vi "Keithley2450 DC Ramp to Block.vi"() -> ()   [LabVIEW 2020]
uses:
  <vilib>/Analysis/1siggen.llb/Ramp Pattern by Samples.vi
  <vilib>/Waveform/WDTOps.llb/WDT Append Waveforms DBL.vi
  <instrlib>/Keithley 2450/Public/Data/Read (Multiple Points).vi
  <vilib>/measure/NI_MAPro.lvlib
  <instrlib>/Keithley 2450/Keithley 2450.lvlib
  <vilib>/Analysis/NI_AALBase.lvlib
panel:
  in  "Source Mode":enum16{"Voltage", "Current"}(ring)=enum."Current"
  in  "VISA resource name":refnum<visa-resource-name>
  in  "Compliance\nVoltage":dbl=210.0
  out "Output Waveform":waveform(dbl)(graph)
  out "Total Time":dbl
  in  "End Amplitude\nHold Time (s)":dbl
  in  "End Amplitude\n(mU)":dbl
  in  "Ramp Rate\n(|mU/s|)":dbl
  in  "Start Amplitude\n(mU)":dbl
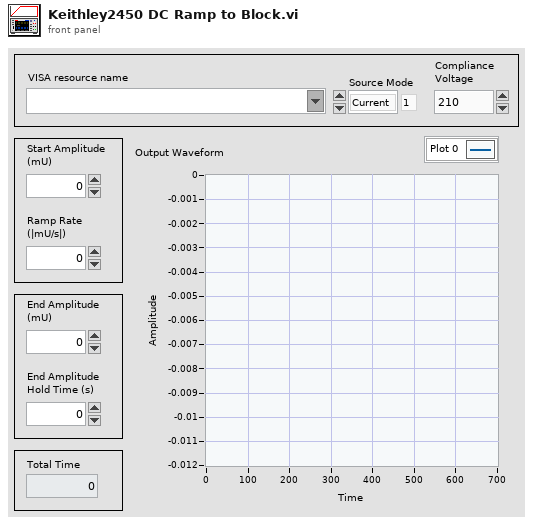
[diagram p1: front panel]
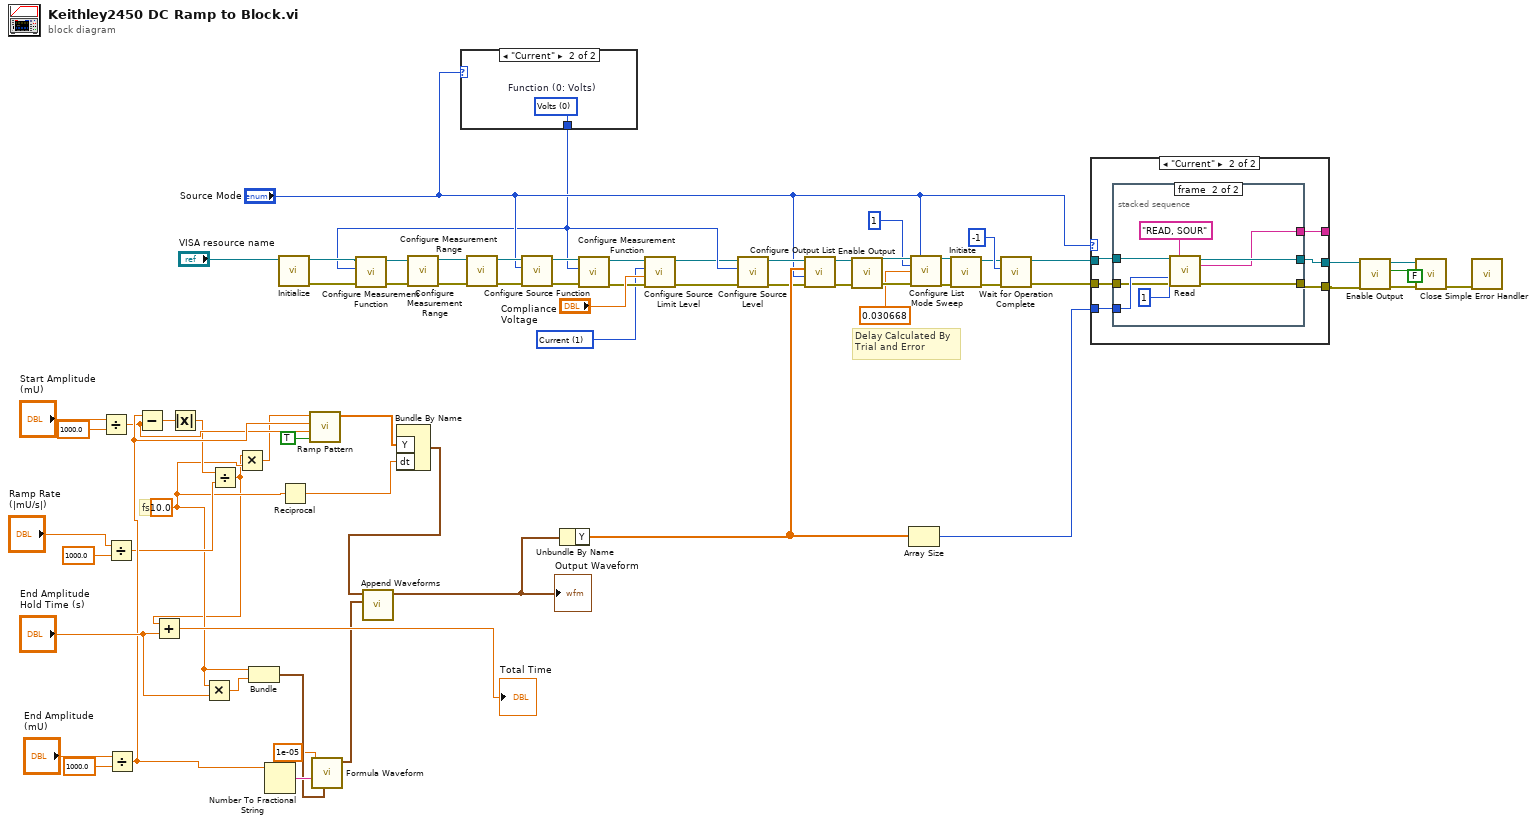
[diagram p0: block diagram]
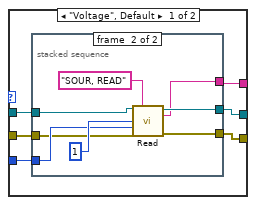
[diagram p2: hidden frame]
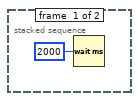
[diagram p3: hidden frame]
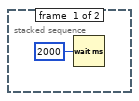
[diagram p4: hidden frame]
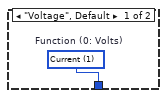
[diagram p5: hidden frame]
diagram:
  w24 = u16 1 items=["Volts", "Current"] ("Function (0: Volts)")
  w2 = 10.0
  # "Delay Calculated By\nTrial and Error"
  # "fs"
  n1 = Divide(x="Start Amplitude\n(mU)", y=1000.0) -> (x/y=w10:dbl)
  n2 = Divide(x="Ramp Rate\n(|mU/s|)", y=1000.0) -> (x/y=w8:dbl)
  n3 = Divide(x="End Amplitude\n(mU)", y=1000.0) -> (x/y=w11:dbl)
  n4 = Subtract(x=w11, y=w10) -> (x-y=w12:dbl)
  n5 = Absolute Value(x=w12) -> (abs(x)=w9:dbl)
  n6 = Multiply(x=w2, y="End Amplitude\nHold Time (s)") -> (x*y=w68:dbl)
  n7 = Divide(x=w9, y=w8) -> (x/y=w1:dbl)
  n8 = Add(x=w1, y="End Amplitude\nHold Time (s)") -> (x+y=→"Total Time":dbl)
  n9 = Multiply(x=w1, y=w2) -> (x*y=w7:dbl)
  n10 = Bundle(w2, w68) -> (w66:cluster{dbl, dbl})  [unwired: 1 in]
  n11 = Number To Fractional String(number=w11) -> (F-format string=w67:string)  [unwired: 3 in]
  n12 = call <instrlib>:"Initialize.vi"("VISA resource name"="VISA resource name") -> ("error out"=w52:errorcluster, "VISA resource name out"=w50:refnum<visa-resource-name>)  [unwired: 9 in]
  n13 = Reciprocal(x=w2) -> (1/x=w5:dbl)
  n14 = call-poly <vilib>:"Ramp Pattern.vi"("exclude end?"=TRUE, "start"=w10, "end"=w11, "samples"=w7) -> ("Ramp Pattern"=w6:dbl[])  [unwired: 6 in, 1 out]
  n15 = call <vilib>:"Formula Waveform.vi"("sampling info"=w66, "formula"=w67, "frequency"=1e-05) -> ("signal out"=w62:waveform(dbl))  [unwired: 7 in, 1 out]
  n16 = Bundle By Name("Y"=w6, "dt"=w5) -> (w4:waveform(dbl))  [unwired: 1 in]
  n17 = call-poly <vilib>:"Append Waveforms.vi"("waveform B"=w62, "waveform A"=w4) -> ("waveform out"=w61:waveform(dbl))  [unwired: 8 in, 1 out]
  "Output Waveform" <- w61
  n18 = case shown="\"Current\"" "Source Mode" {
    tunnel: [w69 w70] -> w25
    frame "Voltage", Default {
      w69 = u16 1 items=["Volts", "Current", "Resistance"]  # Function (0: Volts)
    }
    frame "Current" {
      w70 = u16 0 items=["Volts", "Current", "Resistance"]  # Function (0: Volts)
    }
  }
  n19 = call <instrlib>:"Configure Measurement Function.vi"("error in (no error)"=w52, "Function (0: Volts)"=w25, "VISA resource name"=w50) -> ("error out"=w51:errorcluster, "VISA resource name out"=w49:refnum<visa-resource-name>)  [unwired: 7 in]
  n20 = call <instrlib>:"Configure Measurement Range.vi"("error in (no error)"=w51, "VISA resource name"=w49) -> ("error out"=w60:errorcluster, "VISA resource name out"=w59:refnum<visa-resource-name>)  [unwired: 8 in]
  n21 = call <instrlib>:"Configure Measurement Range.vi"("error in (no error)"=w60, "VISA resource name"=w59) -> ("error out"=w48:errorcluster, "VISA resource name out"=w47:refnum<visa-resource-name>)  [unwired: 8 in]
  n22 = call <instrlib>:"Configure Source Function.vi"("error in (no error)"=w48, "Function (0: Volts)"="Source Mode", "VISA resource name"=w47) -> ("error out"=w35:errorcluster, "VISA resource name out"=w38:refnum<visa-resource-name>)  [unwired: 7 in]
  n23 = Unbundle By Name(w61) -> ("Y"=w33:dbl[])
  n24 = call <instrlib>:"Configure Measurement Function.vi"("error in (no error)"=w35, "Function (0: Volts)"=w25, "VISA resource name"=w38) -> ("error out"=w36:errorcluster, "VISA resource name out"=w37:refnum<visa-resource-name>)  [unwired: 7 in]
  n25 = call <instrlib>:"Configure Source Limit Level.vi"("error in (no error)"=w36, "Source Limit (1.0)"="Compliance\nVoltage", "Function (0: Volts)"=w24, "VISA resource name"=w37) -> ("error out"=w20:errorcluster, "VISA resource name out"=w21:refnum<visa-resource-name>)  [unwired: 6 in]
  n26 = call <instrlib>:"Configure Source Level.vi"("error in (no error)"=w20, "Function (0: Volts)"=w25, "VISA resource name"=w21) -> ("error out"=w29:errorcluster, "VISA resource name out"=w30:refnum<visa-resource-name>)  [unwired: 7 in]
  n27 = call <instrlib>:"Configure Output List.vi"("error in (no error)"=w29, "Source Mode  (0: Voltage)"="Source Mode", "Output List"=w33, "VISA resource name"=w30) -> ("error out"=w55:errorcluster, "VISA resource name out"=w56:refnum<visa-resource-name>)  [unwired: 6 in]
  n28 = call <instrlib>:"Enable Output.vi"("error in (no error)"=w55, "VISA resource name"=w56) -> ("error out"=w46:errorcluster, "VISA resource name out"=w45:refnum<visa-resource-name>)  [unwired: 8 in]
  n29 = Array Size(array=w33) -> (size(s)=w32:i32)
  n30 = call <instrlib>:"Configure List Mode Sweep.vi"("VISA resource name"=w45, "Source Mode  (0: Voltage)"="Source Mode", "Start Index"=u32 1, "Delay (0)"=0.030668, "error in (no error)"=w46) -> ("VISA resource name out"=w43:refnum<visa-resource-name>, "error out"=w42:errorcluster)  [unwired: 9 in]
  n31 = call <instrlib>:"Initiate.vi"("error in (no error)"=w42, "VISA resource name"=w43) -> ("error out"=w40:errorcluster, "VISA resource name out"=w19:refnum<visa-resource-name>)  [unwired: 8 in]
  n32 = call <instrlib>:"Wait for Operation Complete.vi"("error in (no error)"=w40, "Timeout (10000 ms)"=-1, "VISA resource name"=w19) -> ("error out"=w34:errorcluster, "VISA resource name out"=w27:refnum<visa-resource-name>)  [unwired: 7 in]
  n33 = case shown="\"Current\"" "Source Mode" {
    tunnel: [w76 w90] -> w23
    tunnel: [w75 w89] -> w22
    tunnel: w32 -> [w74 w91]
    tunnel: [w73 w88] -> _
    tunnel: w34 -> [w72 w87]
    tunnel: w27 -> [w71 w86]
    frame "Voltage", Default {
      n34 = stacked-sequence {
        tunnel: [_ w85] -> w76
        tunnel: [_ w84] -> w75
        tunnel: [_ w82] -> w73
        tunnel: w74 -> [_ w80]
        tunnel: w72 -> [_ w79]
        tunnel: w71 -> [_ w78]
        frame #0 {
          n35 = Wait (ms)(milliseconds to wait=u32 2000) -> ()  [unwired: 1 out]
        }
        frame #1 {
          n36 = call-poly <instrlib>:"Read.vi"("VISA resource name"=w78, "Buffer Elements"="SOUR, READ", "Start Index (1)"=1, "End Index (1)"=w80, "error in (no error)"=w79) -> ("VISA resource name out"=w85:refnum<visa-resource-name>, "Data out"=w82:string, "error out"=w84:errorcluster)  [unwired: 8 in]
        }
      }
    }
    frame "Current" {
      n37 = stacked-sequence {
        tunnel: [_ w100] -> w90
        tunnel: [_ w99] -> w89
        tunnel: [_ w97] -> w88
        tunnel: w91 -> [_ w95]
        tunnel: w87 -> [_ w94]
        tunnel: w86 -> [_ w93]
        frame #0 {
          n38 = Wait (ms)(milliseconds to wait=u32 2000) -> ()  [unwired: 1 out]
        }
        frame #1 {
          n39 = call-poly <instrlib>:"Read.vi"("VISA resource name"=w93, "Buffer Elements"="READ, SOUR", "Start Index (1)"=1, "End Index (1)"=w95, "error in (no error)"=w94) -> ("VISA resource name out"=w100:refnum<visa-resource-name>, "Data out"=w97:string, "error out"=w99:errorcluster)  [unwired: 8 in]
        }
      }
    }
  }
  n40 = call <instrlib>:"Enable Output.vi"("error in (no error)"=w22, "Enable Output (T: Enable)"=FALSE, "VISA resource name"=w23) -> ("error out"=w54:errorcluster, "VISA resource name out"=w53:refnum<visa-resource-name>)  [unwired: 7 in]
  n41 = call <instrlib>:"Close.vi"("error in (no error)"=w54, "VISA resource name"=w53) -> ("error out"=w57:errorcluster)  [unwired: 9 in]
  n42 = call <vilib>:"Simple Error Handler.vi"("error in (no error)"=w57) -> ()  [unwired: 4 in, 5 out]
